vi "DeviceOn.vi"(8 "error in (no error)":errorcluster, 11 "NHRDCPower in":refnum<class "NHRDCPower.lvclass">) -> (0 "error out":errorcluster, 3 "NHRDCPower out":refnum<class "NHRDCPower.lvclass">)   [LabVIEW 2018, in "AcPwrPlugins.lvlib" / "NHRDCPower.lvclass"]
doc: "This VI enables the instruments output to either generate or recieving a signal."
uses:
  NHRDCPower.lvclass
  <vilib>/ErrorRing/Error Ring.xnode
  <instrlib>/NHRDCPowerModule/NHRDCPowerModule/NHRDCPowerModule.lvlib
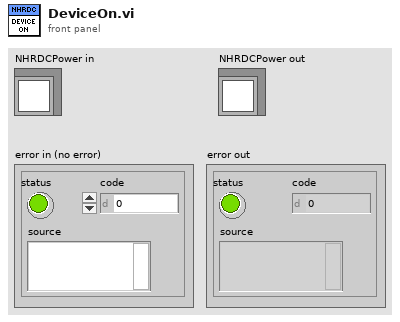
[diagram p1: front panel]
types:
  T1 = typedef "AcPwrPlugins.lvlib/NHRDCPower.lvclass/Modules.ctl" = cluster{"Handle":string, "Name":string, "id query (Yes)":bool, "reset device (Yes)":bool, "Connected":bool, "Initial Battery Detect Voltage (0)":dbl, "SafetySettings":cluster{"SetWatchDog?":bool, "Voltage (V)":dbl, "Current (A)":dbl, "Power (W)":dbl, "Voltage Delay (s)":dbl, "Current Delay (s)":dbl, "Power Delay (s)":dbl}, "Options String":string, "Aperture Time (s)":dbl, "operating state (Off)":i32, "OutputSettings":cluster{"Voltage (V)":dbl, "Current (A)":dbl, "Resistance (Ohms)":dbl, "Power (W)":dbl, "Enable Voltage":bool, "Enable Current":bool, "Enable Resistance":bool, "Enable Power":bool, "Macro After Step Delay  (s)":dbl, "Wait Value (V, A, W)":dbl, "Enable Wait":bool, "Wait on Value":i32}[], "SlewRate":cluster{"Set Voltage Rate V/S":dbl, "Set Current Rate A/S":dbl, "Set Resistance Rate R/S":dbl, "Set Power Rate W/S":dbl}, "Macro":cluster{"Save Macro?":bool, "Load Macro From File?":bool, "Run Macro Continuously?":bool, "Use Macros?":bool, "Load Macro File Path":string, "Save Macro File Path":string}, "Regulation Gain (1=100%)":dbl, "UpdatingOntheFly":bool}[]
  T2 = cluster{"Voltage (V)":dbl, "Current (A)":dbl, "Resistance (Ohms)":dbl, "Power (W)":dbl, "Enable Voltage":bool, "Enable Current":bool, "Enable Resistance":bool, "Enable Power":bool, "Macro After Step Delay  (s)":dbl, "Wait Value (V, A, W)":dbl, "Enable Wait":bool, "Wait on Value":i32}[]
  T3 = cluster{"Voltage (V)":dbl, "Current (A)":dbl, "Resistance (Ohms)":dbl, "Power (W)":dbl, "Enable Voltage":bool, "Enable Current":bool, "Enable Resistance":bool, "Enable Power":bool, "Macro After Step Delay  (s)":dbl, "Wait Value (V, A, W)":dbl, "Enable Wait":bool, "Wait on Value":i32}
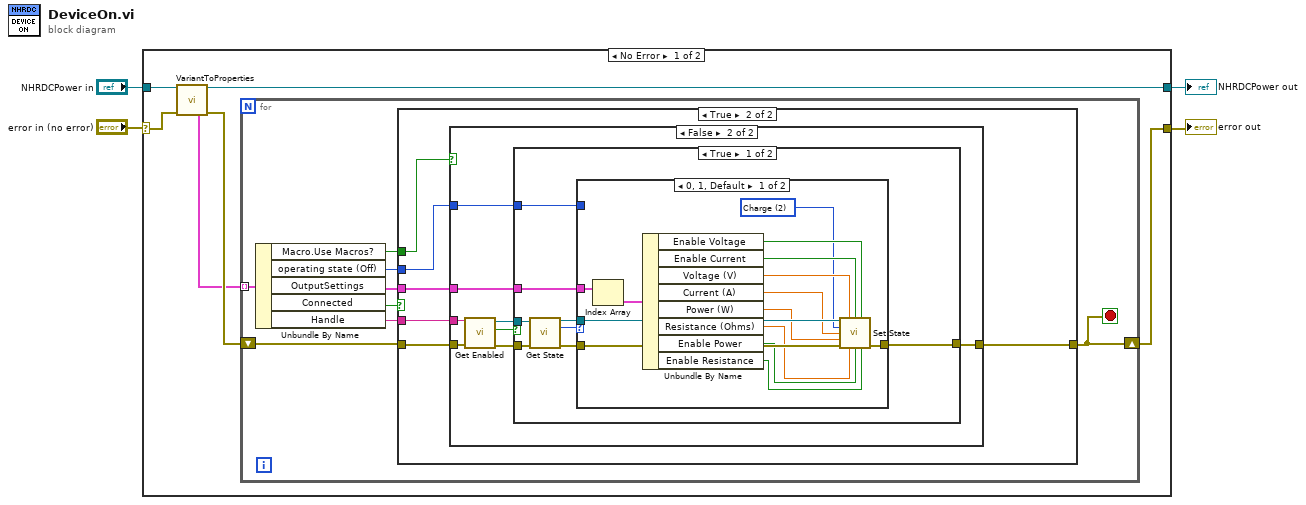
[diagram p0: block diagram]
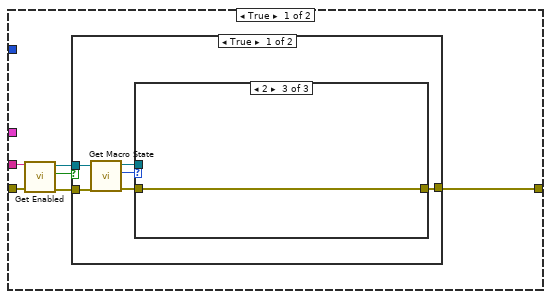
[diagram p3: hidden frame]
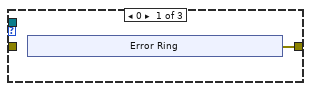
[diagram p4: hidden frame]
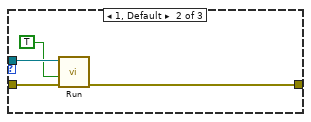
[diagram p5: hidden frame]
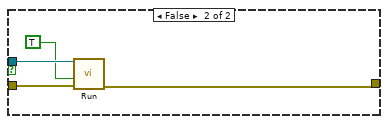
[diagram p6: hidden frame]
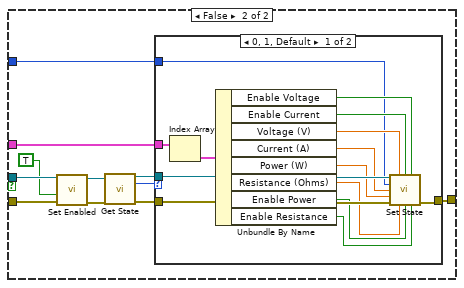
[diagram p8: hidden frame]
diagram:
  n1 = case shown="No Error" "error in (no error)" {
    selector: "error in (no error)" -> [w9 w107]
    tunnel: [w10 w107] -> w1
    tunnel: [w7 w106] -> w3
    tunnel: "NHRDCPower in" -> [w6 w106]
    frame No Error {
      n2 = call "VariantToProperties.vi"("NHRDCPower in"=w6, "error in (no error)"=w9) -> ("NHRDCPower out"=w7:refnum<class "NHRDCPower.lvclass">, "Modules"=w5:T1, "error out"=w8:errorcluster)  [unwired: 7 in, 4 out]
      n3 = for {
        tunnel: w5 -> [w18] mode=indexing
        shift-right: [w16] -> w10
        shift-left: w8 -> [w17]
        stop <- w16 stop-if-true
        n4 = Unbundle By Name(w18) -> ("Macro.Use Macros?"=w11:bool, "operating state (Off)"=w12:i32, "OutputSettings"=w13:T2, "Connected"=w14:bool, "Handle"=w15:string)
        n5 = case shown="True" w14 {
          tunnel: w17 -> [w19 w24]
          tunnel: [w19 w25] -> w16
          tunnel: w15 -> [_ w23]
          tunnel: w13 -> [_ w21]
          tunnel: w12 -> [_ w22]
          tunnel: w11 -> [_ w20]
          frame False {
          }
          frame True {
            n6 = case shown="False" w20 {
              tunnel: [w31 w56] -> w25
              tunnel: w24 -> [w30 w55]
              tunnel: w23 -> [w29 w54]
              tunnel: w22 -> [_ w50]
              tunnel: w21 -> [_ w49]
              frame True {
                n7 = call <instrlib>:"Get Enabled.vi"("error in (no error)"=w30, "instrument handle"=w29) -> ("error out"=w28:errorcluster, "enabled"=w26:bool, "instrument handle out"=w27:refnum<visa-resource-name>)  [unwired: 7 in]
                n8 = case shown="True" w26 {
                  tunnel: [w34 w46] -> w31
                  tunnel: w28 -> [w37 w47]
                  tunnel: w27 -> [w36 w48]
                  frame True {
                    n9 = call <instrlib>:"Get Macro State.vi"("error in (no error)"=w37, "instrument handle"=w36) -> ("error out"=w35:errorcluster, "state"=w32:i32, "instrument handle out"=w33:refnum<visa-resource-name>)  [unwired: 7 in]
                    n10 = case shown="2" w32 {
                      tunnel: w35 -> [_ w43 w44]
                      tunnel: [w38 w40 w44] -> w34
                      tunnel: w33 -> [_ w42 _]
                      frame 0 {
                        n11 = xnode "Error Ring"() -> ("error out"=w38:errorcluster)
                      }
                      frame 1, Default {
                        n12 = call <instrlib>:"Run.vi"("error in (no error)"=w43, "continuous (false)"=TRUE, "instrument handle"=w42) -> ("error out"=w40:errorcluster)  [unwired: 7 in, 1 out]
                      }
                      frame 2 {
                      }
                    }
                  }
                  frame False {
                    n13 = call <instrlib>:"Run.vi"("error in (no error)"=w47, "continuous (false)"=TRUE, "instrument handle"=w48) -> ("error out"=w46:errorcluster)  [unwired: 7 in, 1 out]
                  }
                }
              }
              frame False {
                n14 = call <instrlib>:"Get Enabled.vi"("error in (no error)"=w55, "instrument handle"=w54) -> ("error out"=w53:errorcluster, "enabled"=w51:bool, "instrument handle out"=w52:refnum<visa-resource-name>)  [unwired: 7 in]
                n15 = case shown="True" w51 {
                  tunnel: [w64 w90] -> w56
                  tunnel: w53 -> [w63 w83]
                  tunnel: w52 -> [w62 w84]
                  tunnel: w49 -> [w58 w81]
                  tunnel: w50 -> [w57 w80]
                  frame True {
                    n16 = call <instrlib>:"Get State.vi"("instrument handle"=w62, "error in (no error)"=w63) -> ("instrument handle out"=w59:refnum<visa-resource-name>, "operating state"=w60:i32, "error out"=w61:errorcluster)  [unwired: 3 in, 8 out]
                    n17 = case shown="0, 1, Default" w60 {
                      tunnel: [w77 w79] -> w64
                      tunnel: w61 -> [w78 w79]
                      tunnel: w59 -> [w75 _]
                      tunnel: w58 -> [w76 _]
                      tunnel: w57 -> [_ _]
                      frame 0, 1, Default {
                        w65 = 2 items=["Off", "Stand By", "Charge", "Discharge", "Battery Emulation"] ("operating state (Off)")
                        n18 = Index Array(array=w76) -> (element=w66:T3)  [unwired: 1 in]
                        n19 = Unbundle By Name(w66) -> ("Enable Voltage"=w67:bool, "Enable Current"=w68:bool, "Voltage (V)"=w69:dbl, "Current (A)"=w70:dbl, "Power (W)"=w71:dbl, "Resistance (Ohms)"=w72:dbl, "Enable Power"=w73:bool, "Enable Resistance"=w74:bool)
                        n20 = call <instrlib>:"Set State.vi"("instrument handle"=w75, "voltage (0.0)"=w69, "current enabled (false)"=w68, "voltage enabled (false)"=w67, "operating state (Off)"=w65, "current (0.0)"=w70, "power (0.0)"=w71, "error in (no error)"=w78, "resistance (0.0)"=w72, "power enabled (false)"=w73, "resistance enabled (false)"=w74) -> ("error out"=w77:errorcluster)  [unwired: 3 in, 1 out]
                      }
                      frame 2..4 {
                      }
                    }
                  }
                  frame False {
                    n21 = call <instrlib>:"Set Enabled.vi"("error in (no error)"=w83, "enabled (false)"=TRUE, "instrument handle"=w84) -> ("error out"=w86:errorcluster, "instrument handle out"=w85:refnum<visa-resource-name>)  [unwired: 7 in]
                    n22 = call <instrlib>:"Get State.vi"("instrument handle"=w85, "error in (no error)"=w86) -> ("instrument handle out"=w87:refnum<visa-resource-name>, "operating state"=w88:i32, "error out"=w89:errorcluster)  [unwired: 3 in, 8 out]
                    n23 = case shown="0, 1, Default" w88 {
                      tunnel: [w103 w105] -> w90
                      tunnel: w89 -> [w104 w105]
                      tunnel: w87 -> [w102 _]
                      tunnel: w81 -> [w93 _]
                      tunnel: w80 -> [w91 _]
                      frame 0, 1, Default {
                        n24 = Index Array(array=w93) -> (element=w92:T3)  [unwired: 1 in]
                        n25 = Unbundle By Name(w92) -> ("Enable Voltage"=w94:bool, "Enable Current"=w95:bool, "Voltage (V)"=w96:dbl, "Current (A)"=w97:dbl, "Power (W)"=w98:dbl, "Resistance (Ohms)"=w99:dbl, "Enable Power"=w100:bool, "Enable Resistance"=w101:bool)
                        n26 = call <instrlib>:"Set State.vi"("instrument handle"=w102, "voltage (0.0)"=w96, "current enabled (false)"=w95, "voltage enabled (false)"=w94, "operating state (Off)"=w91, "current (0.0)"=w97, "power (0.0)"=w98, "error in (no error)"=w104, "resistance (0.0)"=w99, "power enabled (false)"=w100, "resistance enabled (false)"=w101) -> ("error out"=w103:errorcluster)  [unwired: 3 in, 1 out]
                      }
                      frame 2..4 {
                      }
                    }
                  }
                }
              }
            }
          }
        }
      }
    }
    frame Error {
    }
  }
  "error out" <- w1
  "NHRDCPower out" <- w3
